vi "Get GUIDs from Custom Device XML.vi"(7 "error in":errorcluster, 10 "CustomDevice in":refnum<k24>) -> (0 "error out":errorcluster, 2 "set out":set{string}(c389), 3 "CustomDevice out":refnum<k24>)   [LabVIEW 2020, in "Utility.lvlib"]
uses:
  Utility.lvlib
  NationalInstruments.VeriStand.XMLReader
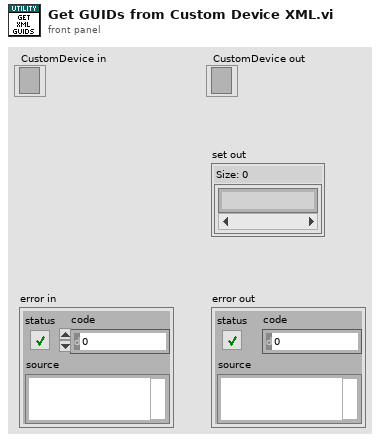
[diagram p1: front panel]
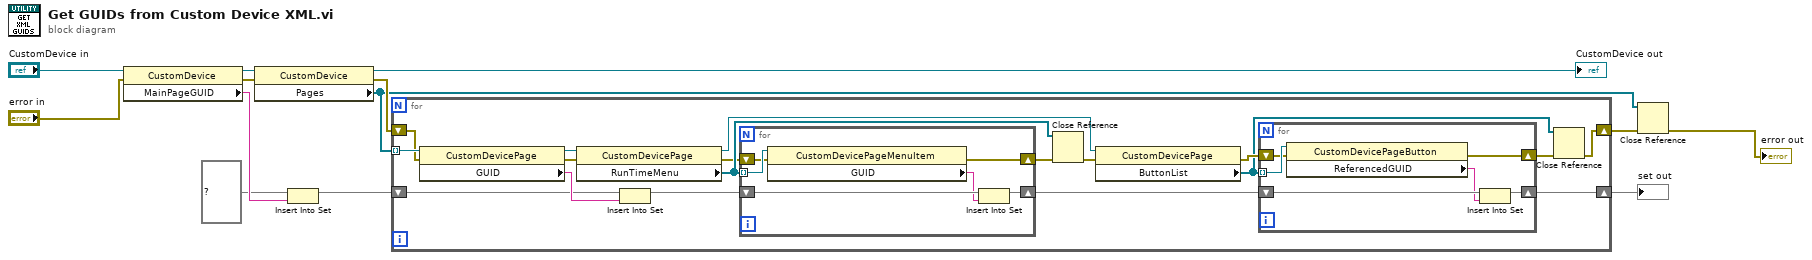
[diagram p0: block diagram]
diagram:
  n1 = property class="CustomDevice"(reference="CustomDevice in", error in="error in") -> (reference out=w9:refnum<k24>, error out=w5:errorcluster, "MainPageGUID"=w13:string)
  n2 = property class="CustomDevice"(reference=w9, error in=w5) -> (reference out=→"CustomDevice out":refnum<k24>, error out=w4:errorcluster, "Pages"=w2:refnum<k24>[])
  n3 = Insert Into Set(10:w13, 11:set{string} {} ("set in")) -> (3:w12:set{string})  [unwired: 1 out]
  n4 = for {
    tunnel: w2 -> [w31] mode=indexing
    shift-right: [w24] -> w10
    shift-left: w12 -> [w27]
    shift-right: [w15] -> w3
    shift-left: w4 -> [w23]
    n5 = property class="CustomDevicePage"(reference=w31, error in=w23) -> (reference out=w30:refnum<k24>, error out=w22:errorcluster, "GUID"=w28:string)
    n6 = property class="CustomDevicePage"(reference=w30, error in=w22) -> (reference out=w29:refnum<k24>, error out=w18:errorcluster, "RunTimeMenu"=w20:refnum<k24>[])
    n7 = Insert Into Set(10:w28, 11:w27) -> (3:w26:set{string})  [unwired: 1 out]
    n8 = for {
      tunnel: w20 -> [w43] mode=indexing
      shift-right: [w41] -> w25
      shift-left: w26 -> [w42]
      shift-right: [w39] -> w19
      shift-left: w18 -> [w38]
      n9 = property class="CustomDevicePageMenuItem"(reference=w43, error in=w38) -> (error out=w39:errorcluster, "GUID"=w40:string)  [unwired: 1 out]
      n10 = Insert Into Set(10:w40, 11:w42) -> (3:w41:set{string})  [unwired: 1 out]
    }
    n11 = Close Reference(reference=w20, error in (no error)=w19) -> (error out=w21:errorcluster)
    n12 = property class="CustomDevicePage"(reference=w29, error in=w21) -> (error out=w17:errorcluster, "ButtonList"=w14:refnum<k24>[])  [unwired: 1 out]
    n13 = for {
      tunnel: w14 -> [w37] mode=indexing
      shift-right: [w35] -> w24
      shift-left: w25 -> [w36]
      shift-right: [w32] -> w16
      shift-left: w17 -> [w33]
      n14 = property class="CustomDevicePageButton"(reference=w37, error in=w33) -> (error out=w32:errorcluster, "ReferencedGUID"=w34:string)  [unwired: 1 out]
      n15 = Insert Into Set(10:w34, 11:w36) -> (3:w35:set{string})  [unwired: 1 out]
    }
    n16 = Close Reference(reference=w14, error in (no error)=w16) -> (error out=w15:errorcluster)
  }
  "set out" <- w10
  n17 = Close Reference(reference=w2, error in (no error)=w3) -> (error out=→"error out":errorcluster)
